vi "Refresh Dashboard.vi"(7 "Num Col":i16, 10 "appended array":string[](array[string]), 11 "Refnum in":refnum<k1>) -> (3 "Array":T1(array[cluster]))   [LabVIEW 2020, in "CSM-TagDashboard.lvlib"]
uses:
  CSM-TagDashboard.lvlib
  6bf5eeed-4598-4c59-888d-74909260dc4d.vi
  bd4fe9ea-d1ec-4222-8a83-7b7899176eaf.vi
  fc032499-1e43-4e1f-b8eb-a35f5c7ea8a4.vi
  510f4942-93b2-494c-912b-5c852fd46c70.vi
  <userlib>/_NEVSTOP/TagDB/_Support/Error/_[error50000]Invalid DB REF.vi
  <userlib>/_NEVSTOP/TagDB/_Support/DataAccess/TagDB Ref to DVR.vi
  <userlib>/_NEVSTOP/TagDB/_Support/DataAccess/_NameCacher.vi
  <userlib>/_NEVSTOP/TagDB/_Support/Error/_[error50002]Invalid DataType.vi
  <userlib>/_NEVSTOP/TagDB/_Support/URL/TRIM-BOTH-SPACE.vi
  <userlib>/_NEVSTOP/TagDB/_Support/Error/_Build Error Cluster.vi
  <userlib>/_NEVSTOP/TagDB/TagDB.lvlib
  ecca9915-5b08-49b8-9981-7a1368530b08.vi
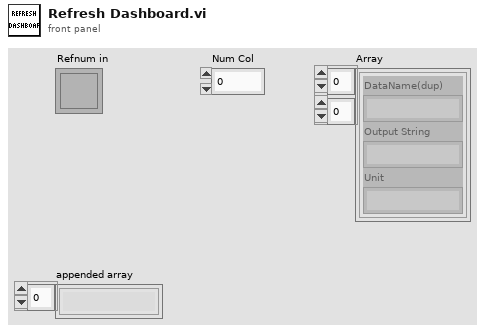
[diagram p1: front panel]
types:
  T1 = cluster{"DataName(dup)":string, "Output String":string, "Unit":string}[][]
  T2 = cluster{"DataName(dup)":string, "Data":string, "Unit":string}[][]
  T3 = cluster{"DataName(dup)":string, "Format String":string, "Format String":string}
  T4 = cluster{"DataName(dup)":string, "Data":string, "Unit":string}
  T5 = cluster{"DataName(dup)":string, "Format String":string, "Format String":string}[][]
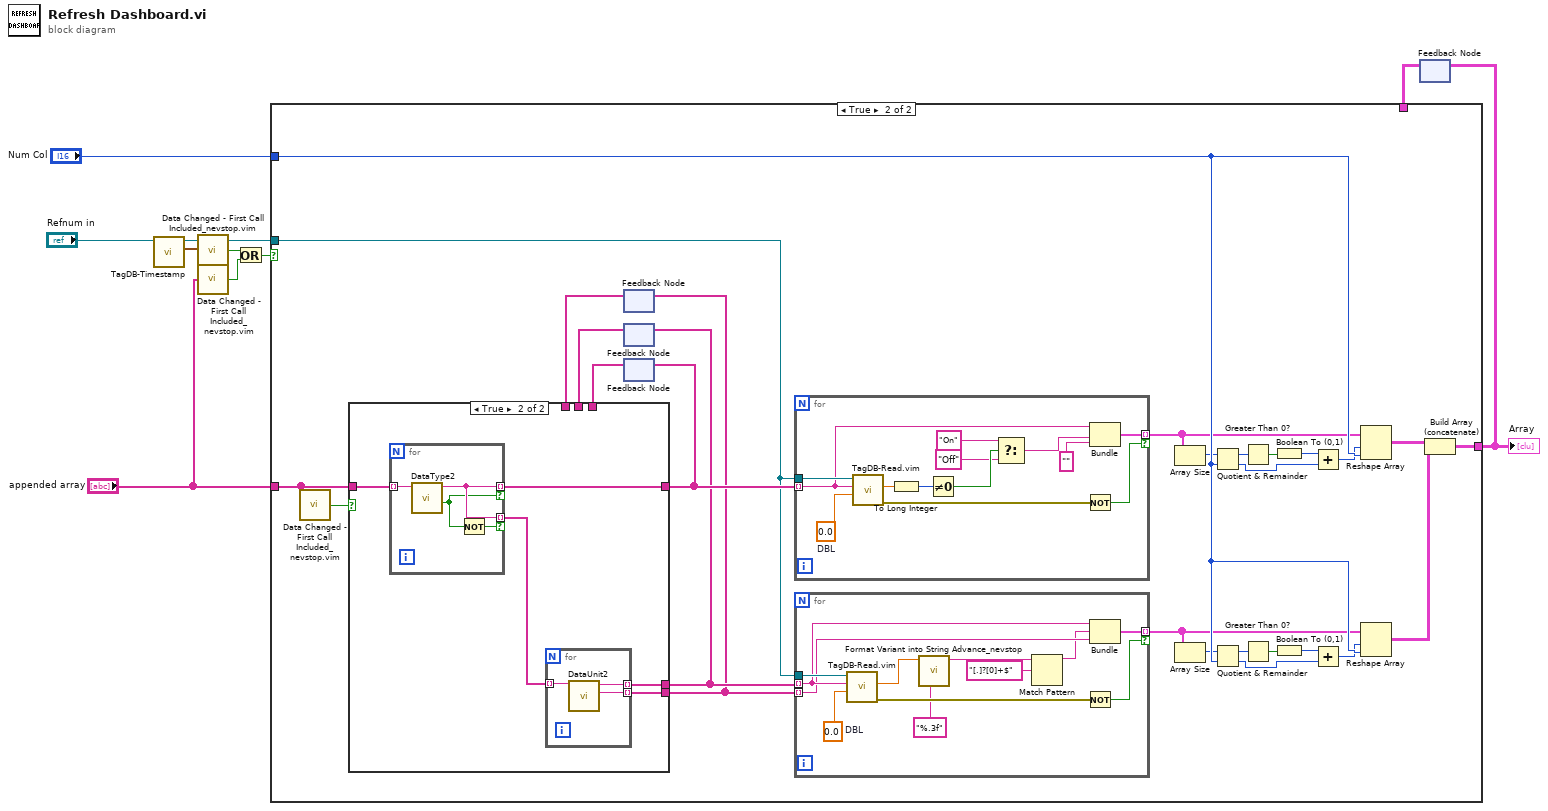
[diagram p0: block diagram]
diagram:
  n1 = call <userlib>:"TagDB-Timestamp.vi"("DB Ref"="Refnum in") -> ("Global Change Timestamp"=w7:timestamp, "DB Ref (dup)"=w8:refnum<k1>)  [unwired: 7 in, 2 out]
  n2 = call "Data Changed - First Call Included_nevstop.vim"("Variant"=w7) -> ("Changed"=w6:bool)
  n3 = call "Data Changed - First Call Included_nevstop.vim"("Variant"="appended array") -> ("Changed"=w1:bool)
  n4 = Or(x=w6, y=w1) -> (x .or. y?=w2:bool)
  n5 = feedback #1() -> (w4:T2)  [unwired: 1 in]
  n6 = case shown="True" w2 {
    tunnel: [w11 w38] -> w5
    tunnel: "Num Col" -> [_ w35]
    tunnel: "appended array" -> [_ w20]
    tunnel: w8 -> [_ w16]
    tunnel: w4 -> [w11 _]
    frame False {
    }
    frame True {
      n7 = call "Data Changed - First Call Included_nevstop.vim"("Variant"=w20) -> ("Changed"=w19:bool)
      n8 = feedback #2() -> (w12:string[])  [unwired: 1 in]
      n9 = feedback #3() -> (w14:string[])  [unwired: 1 in]
      n10 = feedback #4() -> (w17:string[])  [unwired: 1 in]
      n11 = case shown="True" w19 {
        tunnel: [w39 w46] -> w13
        tunnel: [w40 w45] -> w15
        tunnel: [w41 w43] -> w18
        tunnel: w20 -> [_ w42]
        tunnel: w17 -> [w41 _]
        tunnel: w14 -> [w40 _]
        tunnel: w12 -> [w39 _]
        frame False {
        }
        frame True {
          n12 = for {
            tunnel: w42 -> [w53] mode=indexing
            tunnel: [w52] -> w43 mode=indexing if=w51
            tunnel: [w52] -> w44 mode=indexing if=w50
            n13 = call "DataType2.vi"("DataName"=w53) -> ("isBool?"=w51:bool, "DataName(dup)"=w52:string)  [unwired: 8 in, 1 out]
            n14 = Not(x=w51) -> (.not. x?=w50:bool)
          }
          n15 = for {
            tunnel: w44 -> [w49] mode=indexing
            tunnel: [w48] -> w45 mode=indexing
            tunnel: [w47] -> w46 mode=indexing
            n16 = call "DataUnit2.vi"("DataName"=w49) -> ("Unit"=w47:string, "DataName(dup)"=w48:string)  [unwired: 9 in]
          }
        }
      }
      n17 = feedback-in #2(w13) -> ()
      n18 = feedback-in #3(w15) -> ()
      n19 = feedback-in #4(w18) -> ()
      n20 = for {
        tunnel: [w73] -> w34 mode=indexing if=w78
        tunnel: w16 -> [w77]
        tunnel: w18 -> [w75] mode=indexing
        w76 = 0.0  # DBL
        n21 = call "TagDB-Read.vim"("Type(empty to read as variant)"=w76, "name"=w75, "TagDB"=w77) -> ("error out"=w71:errorcluster, "Value"=w72:dbl)  [unwired: 3 in, 4 out]
        n22 = To Long Integer(number=w72) -> (32bit integer=w70:i32)
        n23 = Not Equal To 0?(x=w70) -> (x != 0?=w69:bool)
        n24 = Select(t="On" ("Format String"), s=w69, f="Off" ("Format String")) -> (s? t:f=w66:string)
        n25 = Not(x=w71) -> (.not. x?=w78:bool)
        n26 = Bundle("DataName(dup)"=w75, "Format String"=w66, "Format String"="") -> (w73:T3)  [unwired: 1 in]
      }
      n27 = for {
        tunnel: [w61] -> w33 mode=indexing if=w65
        tunnel: w16 -> [w64]
        tunnel: w15 -> [w62] mode=indexing
        tunnel: w13 -> [w57] mode=indexing
        w63 = 0.0  # DBL
        n28 = call "TagDB-Read.vim"("Type(empty to read as variant)"=w63, "name"=w62, "TagDB"=w64) -> ("error out"=w60:errorcluster, "Value"=w59:dbl)  [unwired: 3 in, 4 out]
        n29 = call <userlib>:"Format Variant into String Advance_nevstop.vi"("Format String"="%.3f", "Variant"=w59) -> ("Data"=w56:string)  [unwired: 7 in, 2 out]
        n30 = Match Pattern(string=w56, regular expression="[.]?[0]+$") -> (before substring=w55:string)  [unwired: 1 in, 3 out]
        n31 = Not(x=w60) -> (.not. x?=w65:bool)
        n32 = Bundle("DataName(dup)"=w62, "Data"=w55, "Unit"=w57) -> (w61:T4)  [unwired: 1 in]
      }
      n33 = Array Size(array=w34) -> (size(s)=w27:i32)
      n34 = Array Size(array=w33) -> (size(s)=w26:i32)
      n35 = Quotient & Remainder(x=w27, y=w35) -> (x-y*floor(x/y)=w28:i32, floor(x/y)=w32:i32)
      n36 = Quotient & Remainder(x=w26, y=w35) -> (x-y*floor(x/y)=w25:i32, floor(x/y)=w21:i32)
      n37 = Greater Than 0?(x=w28) -> (x > 0?=w29:bool)
      n38 = Greater Than 0?(x=w25) -> (x > 0?=w24:bool)
      n39 = Boolean To (0,1)(Boolean=w29) -> (0, 1=w31:i16)
      n40 = Boolean To (0,1)(Boolean=w24) -> (0, 1=w22:i16)
      n41 = Add(x=w31, y=w32) -> (x+y=w30:i32)
      n42 = Add(x=w22, y=w21) -> (x+y=w23:i32)
      n43 = Reshape Array(w34, w30, w35) -> (w36:T5)
      n44 = Reshape Array(w33, w23, w35) -> (w37:T2)
      n45 = Build Array (concatenate)(w36, w37) -> (w38:T2)
    }
  }
  "Array" <- w5
  n46 = feedback-in #1(w5) -> ()
